vi "ConfigSampleMode.vi"(8 "error in (no error)":errorcluster, 11 "DigitizerBase in":refnum<class "DigitizerBase.lvclass">) -> (0 "error out":errorcluster, 3 "DigitizerBase out":refnum<class "DigitizerBase.lvclass">)   [LabVIEW 2014, in "DigitizerPlugins.lvlib" / "DigitizerBase.lvclass"]
uses:
  DigitizerBase.lvclass
  DigitizerBase.lvclass/DigitizerBase.ctl
  Accessors/Read InstRef.vi
  Accessors/Read Acquisition.vi
  Accessors/Write InstRef.vi
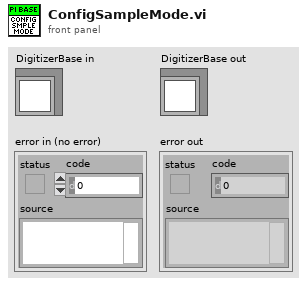
[diagram p1: front panel]
types:
  T1 = typedef "DigitizerPlugins.lvlib/DigitizerBase.lvclass/Acquisition.ctl" = cluster{"SampleRate":dbl, "RecordSize":i32, "NumRecords":i32, "SampleMode":i32, "Timeout (ms)":i32}
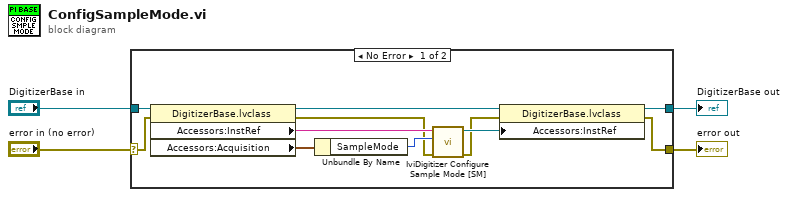
[diagram p0: block diagram]
diagram:
  n1 = case shown="No Error" "error in (no error)" {
    selector: "error in (no error)" -> [w12 w17]
    tunnel: [w5 w17] -> w3
    tunnel: [w8 w16] -> w1
    tunnel: "DigitizerBase in" -> [w15 w16]
    frame No Error {
      n2 = property class="DigitizerBase.lvclass"(reference=w15, error in=w12) -> (reference out=w14:refnum<class "DigitizerBase.lvclass">, error out=w9:errorcluster, "Accessors:InstRef"=w13:string, "Accessors:Acquisition"=w11:T1)
      n3 = Unbundle By Name(w11) -> ("SampleMode"=w10:i32)
      n4 = call <vilib>:"IviDigitizer Configure Sample Mode [SM].vi"("error in (no error)"=w9, "Sample Mode (Real Time)"=w10, "instrument handle"=w13) -> ("error out"=w6:errorcluster, "instrument handle out"=w7:refnum<k15>)  [unwired: 7 in]
      n5 = property class="DigitizerBase.lvclass"(reference=w14, error in=w6, "Accessors:InstRef"=w7) -> (reference out=w8:refnum<class "DigitizerBase.lvclass">, error out=w5:errorcluster)
    }
    frame Error {
    }
  }
  "error out" <- w3
  "DigitizerBase out" <- w1
